vi "uintInRangeCoerceELowerEUpper.vi"(8 "Error in (no error)":errorcluster, 9 "Lowerlimit":refnum<class "UintClass.lvclass">, 10 "Int in":refnum<class "UintClass.lvclass">, 11 "Upperlimit":refnum<class "UintClass.lvclass">) -> (0 "Error out":errorcluster, 1 "Timing":u32, 2 "In Range?":bool, 3 "Coerced(Int)":refnum<class "UintClass.lvclass">)   [LabVIEW 2011, in "UintClass.lvclass"]
uses:
  UintClass.lvclass
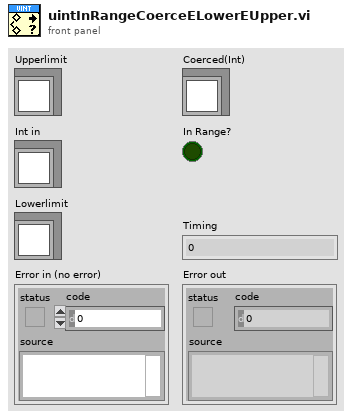
[diagram p1: front panel]
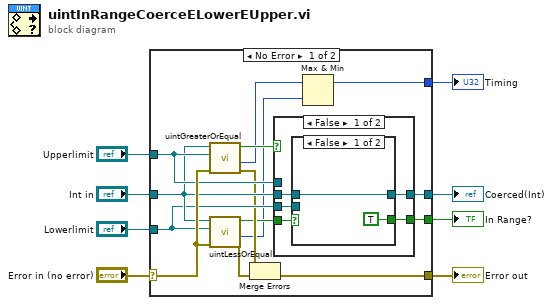
[diagram p0: block diagram]
diagram:
  n1 = case shown="No Error" "Error in (no error)" {
    selector: "Error in (no error)" -> [w22 w32]
    tunnel: "Upperlimit" -> [w20 _]
    tunnel: "Int in" -> [w19 _]
    tunnel: "Lowerlimit" -> [w18 _]
    tunnel: [w15 w32] -> w4
    tunnel: [w14 _] -> w3
    tunnel: [w10 _] -> w2
    tunnel: [w9 _] -> w1
    frame No Error {
      n2 = call "uintGreaterOrEqual.vi"("Error in (no error)"=w22, "Int2 in"=w20, "Int1 in"=w19) -> ("Error out"=w17:errorcluster, "Timing"=w12:u32, "Int1 >= Int2?"=w21:bool)  [unwired: 6 in]
      n3 = call "uintLessOrEqual.vi"("Error in (no error)"=w22, "Int2 in"=w18, "Int1 in"=w19) -> ("Error out"=w16:errorcluster, "Timing"=w11:u32, "Int1 <= Int2?"=w13:bool)  [unwired: 6 in]
      n4 = Merge Errors(w17, w16) -> (w15:errorcluster)
      n5 = case shown="False" w21 {
        tunnel: w20 -> [_ w31]
        tunnel: w19 -> [w26 _]
        tunnel: w18 -> [w25 _]
        tunnel: [w24 w31] -> w14
        tunnel: w13 -> [w27 _]
        tunnel: [w23 _] -> w9
        frame False {
          n6 = case shown="False" w27 {
            tunnel: w26 -> [w29 _]
            tunnel: w25 -> [_ w30]
            tunnel: [w29 w30] -> w24
            tunnel: [TRUE ("In Range?") _] -> w23
            frame False {
            }
            frame True {
            }
          }
        }
        frame True {
        }
      }
      n7 = Max & Min(x=w12, y=w11) -> (max(x,y)=w10:u32)  [unwired: 1 out]
    }
    frame Error {
    }
  }
  "Error out" <- w4
  "In Range?" <- w1
  "Coerced(Int)" <- w3
  "Timing" <- w2
